vi "Find Acyclic Frame Section.vi"(8 "error in":errorcluster, 11 "bus controller in":T1 format="%.0x") -> (0 "error out":errorcluster, 2 "acyclic frames section":T1 format="%.0x", 3 "bus controller out":T1 format="%.0x", 4 "found?":bool)   [LabVIEW 2020, in "AIM MIL-STD-1553 Scripting.lvlib"]
doc: "Within the specified <b>port in</b>, searches for an instance of a bus controller. If a bus controller is found, returns the <b>bus controller</b> reference. If no bus controller is found, the returned reference is invalid and <b>found?</b> equals False."
uses:
  AIM MIL-STD-1553 Scripting.lvlib
  <vilib>/NI VeriStand/Custom Device API/Custom Device Item Ref.ctl
  Constants.vi
  <vilib>/NI VeriStand/Custom Device Tools/Custom Device Utility Library/NI VeriStand - Search for Item by GUID.vi
  <vilib>/NI VeriStand/Custom Device Tools/Custom Device Utility Library/Custom Device Utility Library.lvlib
  <vilib>/NI VeriStand/Custom Device API/Custom Device API.lvlib
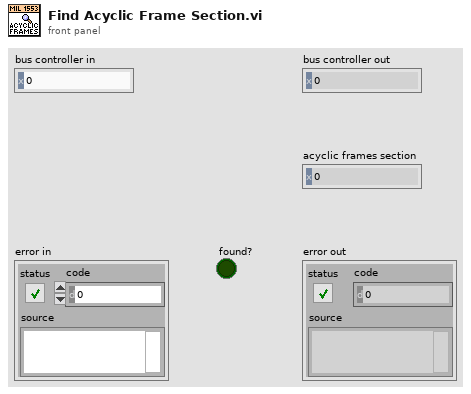
[diagram p1: front panel]
types:
  T1 = typedef "Custom Device API.lvlib/Custom Device Item Ref.ctl" = u64
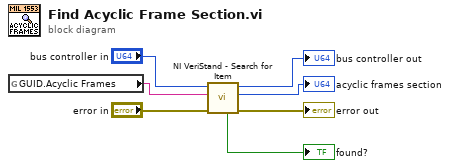
[diagram p0: block diagram]
diagram:
  n1 = global read "Constants.vi" "GUID.Acyclic Frames"() -> (w7:string)
  n2 = call-poly <vilib>:"NI VeriStand - Search for Item.vi"("error in"="error in", "Item GUID"=w7, "Section Ref in"="bus controller in") -> ("error out"=→"error out":errorcluster, "Item Ref"=→"acyclic frames section":T1, "Section Ref out"=→"bus controller out":T1, "Found"=→"found?":bool)  [unwired: 5 in]
